vi "ModifyChnlHW.vi"(8 "error in (no error)":errorcluster, 11 "BME_DG_G08_Chnl in":refnum<class "BME_DG_G08_Chnl.lvclass">) -> (0 "error out":errorcluster, 3 "BME_DG_G08_Chnl out":refnum<class "BME_DG_G08_Chnl.lvclass">)   [LabVIEW 2009, in "POLARIS BME DG.lvlib" / "BME_DG_G08_Chnl.lvclass"]
doc: "This VI calls DLL Set_G08_Delay\n\nATTENTION: it causes asyncronouse HW parameter change. It may be good idea to deactivate some HW before or use synchronus parameter change mechanism in case of SG08P2.\n\n\nlast change 201211-08: course output offset added. course ouput value must be \n=outputmodulo - 1, other wise channel fires one trigger to late.\n\n---------------\n\nauthor: Alexander Kessler, Helmholtz-Institut-Jena \nmaintainer: Alexander Kessler: alexander.kessler@uni-jena.de\n\n\nLicense Agreement for this software:\n\nCopyright (C)\nHelmholtz-Institut-Jena\nFröbelsteg 3\n07743 Jena\nGermany\n\nContact: alexander.kessler@uni-jena.de\n\nThis program is free software; you can redistribute it and/or modify it under the terms of the GNU General Public License as published by the Free Software Foundation; either version 2 of the license, or (at your option) any later version.\n\nThis program is distributed in the hope that it will be useful, but WITHOUT ANY WARRANTY; without even the implied warranty of MERCHANTABILITY or FITNESS FOR A PARTICULAR PURPOSE. See the GNU General License for more details (http://www.gnu.org)."
uses:
  BME_DG_G08_Chnl.lvclass
  BME_DG_G08_Chnl.lvclass/BME_DG_G08_Chnl.ctl
  POLARIS BME DG.lvlib
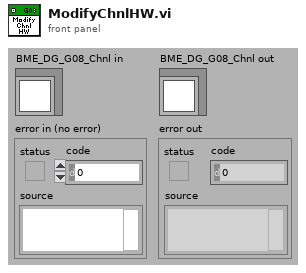
[diagram p1: front panel]
types:
  T1 = cluster{"Channel":u32, "Fire First (µs)":dbl, "Pulse Width (µs)":dbl, "Output Modulo":u32, "Output Offset":u32, "Go Signal":u32, "Polarity":bool, "Terminate":bool, "Disconnect (E,F)":bool, "Onto MsBus (E,F)":bool, "Input Positive (E,F)":bool}
  T2 = typedef "POLARIS BME DG.lvlib/ChnlSettings.ctl" = cluster{" Delay (µs)":dbl, "On?":bool, "PositiveVoltage?":bool, "50OhmTerminated? ":bool, "25OhmOutput?":bool}
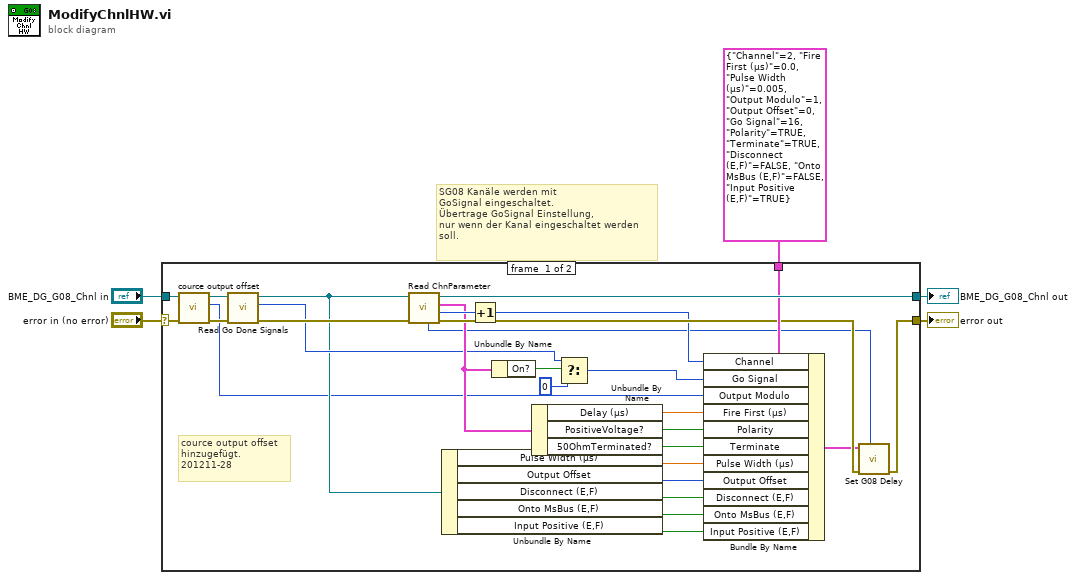
[diagram p0: block diagram]
diagram:
  # "SG08 Kanäle werden mit \nGoSignal eingeschaltet.\nÜbertrage GoSignal Einstellung,\nnur wenn der Kanal eingeschaltet werden\nsoll."
  n1 = case shown="No Error" "error in (no error)" {
    selector: "error in (no error)" -> [w8 w35]
    tunnel: [w12 w35] -> w2
    tunnel: [w33 w34] -> w4
    tunnel: "BME_DG_G08_Chnl in" -> [w10 w34]
    tunnel: T1 {"Channel"=2, "Fire First (µs)"=0.0, "Pulse Width (µs)"=0.005, "Output Modulo"=1, "Output Offset"=0, "Go Signal"=16, "Polarity"=TRUE, "Terminate"=TRUE, "Disconnect (E,F)"=FALSE, "Onto MsBus (E,F)"=FALSE, "Input Positive (E,F)"=TRUE} ("Settings") -> [w32 _]
    frame #0 {
      # "cource output offset\nhinzugefügt.\n201211-28"
      n2 = call-dynamic "cource output offset.vi"("error in (no error)"=w8, "BME_DG_G08_Chnl in"=w10) -> ("error out"=w7:errorcluster, "OutputModulo"=w6:i32, "BME_DG_G08_Chnl out"=w9:refnum<class "BME_DG_G08_Chnl.lvclass">)  [unwired: 6 in, 1 out]
      n3 = call-dynamic "Read Go Done Signals.vi"("error in (no error)"=w7, "BME_DG_G05P2_Chnl in"=w9) -> ("error out"=w23:errorcluster, "Go Signal"=w18:u32, "BME_DG_G05P2_Chnl out"=w11:refnum<class "BME_DG_G08_Chnl.lvclass">)  [unwired: 6 in, 1 out]
      n4 = call-dynamic "Read ChnParameter.vi"("error in (no error)"=w23, "BME_DG_Chnl in"=w11) -> ("error out"=w31:errorcluster, "Nr"=w30:i32, "ChnParemater"=w20:T2, "BME_DG_Chnl out"=w33:refnum<class "BME_DG_G08_Chnl.lvclass">, "DG Nr"=w13:i32)  [unwired: 4 in, 1 out]
      n5 = Unbundle By Name(w11) -> ("Pulse Width (µs)"=w28:dbl, "Output Offset"=w27:u32, "Disconnect (E,F)"=w26:bool, "Onto MsBus (E,F)"=w25:bool, "Input Positive (E,F)"=w24:bool)
      n6 = Increment(x=w30) -> (x+1=w15:i32)
      n7 = Unbundle By Name(w20) -> ("On?"=w19:bool)
      n8 = Unbundle By Name(w20) -> ("Delay (µs)"=w29:dbl, "PositiveVoltage?"=w22:bool, "50OhmTerminated?"=w21:bool)
      n9 = Select(t=w18, s=w19, f=u32 0) -> (s? t:f=w16:u32)
      n10 = Bundle By Name(cluster=w32, "Channel"=w15, "Go Signal"=w16, "Output Modulo"=w6, "Fire First (µs)"=w29, "Polarity"=w22, "Terminate"=w21, "Pulse Width (µs)"=w28, "Output Offset"=w27, "Disconnect (E,F)"=w26, "Onto MsBus (E,F)"=w25, "Input Positive (E,F)"=w24) -> (w14:T1)
      n11 = call "Set G08 Delay.vi"("DG Number"=w13, "error in (no error)"=w31, "Settings"=w14) -> ("error out"=w12:errorcluster)  [unwired: 8 in]
    }
    frame #1 {
    }
  }
  "error out" <- w2
  "BME_DG_G08_Chnl out" <- w4
